vi "Error Interpreter.vi"(0 "request packet":string, 1 "response packet":string, 2 "packet type":T1(ring), 3 "error in (no error)":errorcluster) -> (10 "error out":errorcluster)   [LabVIEW 2024, in "OptoMMP.lvlib"]
doc: "Takes an OptoMMP hexadecimal string formatted response packet of any type, locates the rcode, and outputs a corresponding error code and message. If there is a TCP read error, an Opto error will not be returned.\n\nLast updated: 7/17/2025"
uses:
  <instrlib>/OptoMMP/OptoMMP.lvlib
panel:
  # "Copyright (c) 2025 California Institute of Technology (Caltech).\nU.S. Government sponsorship acknowledged.\n\nLicensed under the Apache License, Version 2.0 (the \"License\");\nyou may not use this file except in compliance with the License.\nYou may obtain a copy of the License at\n\n    http://www.apache.org/licenses/LICENSE-2.0\n\nUnless required by applicable law or agreed to in writing, software\ndistributed under the License is distributed on an \"AS IS\" BASIS,\nWITHOUT WARRANTIES OR CONDITIONS OF ANY KIND, either express or implied.\nSee the License for the specific language governing permissions and\nlimitations under the License."
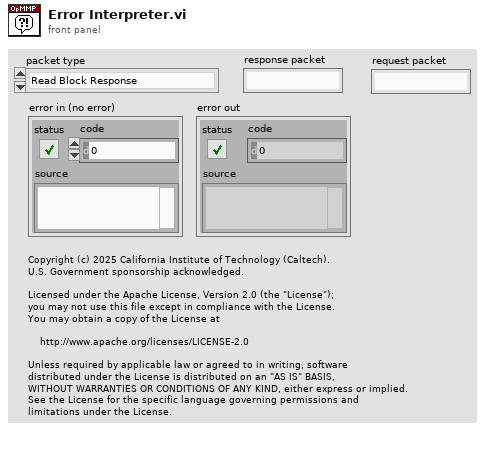
[diagram p1: front panel]
types:
  T1 = enum16{"Read Block Response", "Write Quadlet or Block Response", "Read Quadlet Response"}
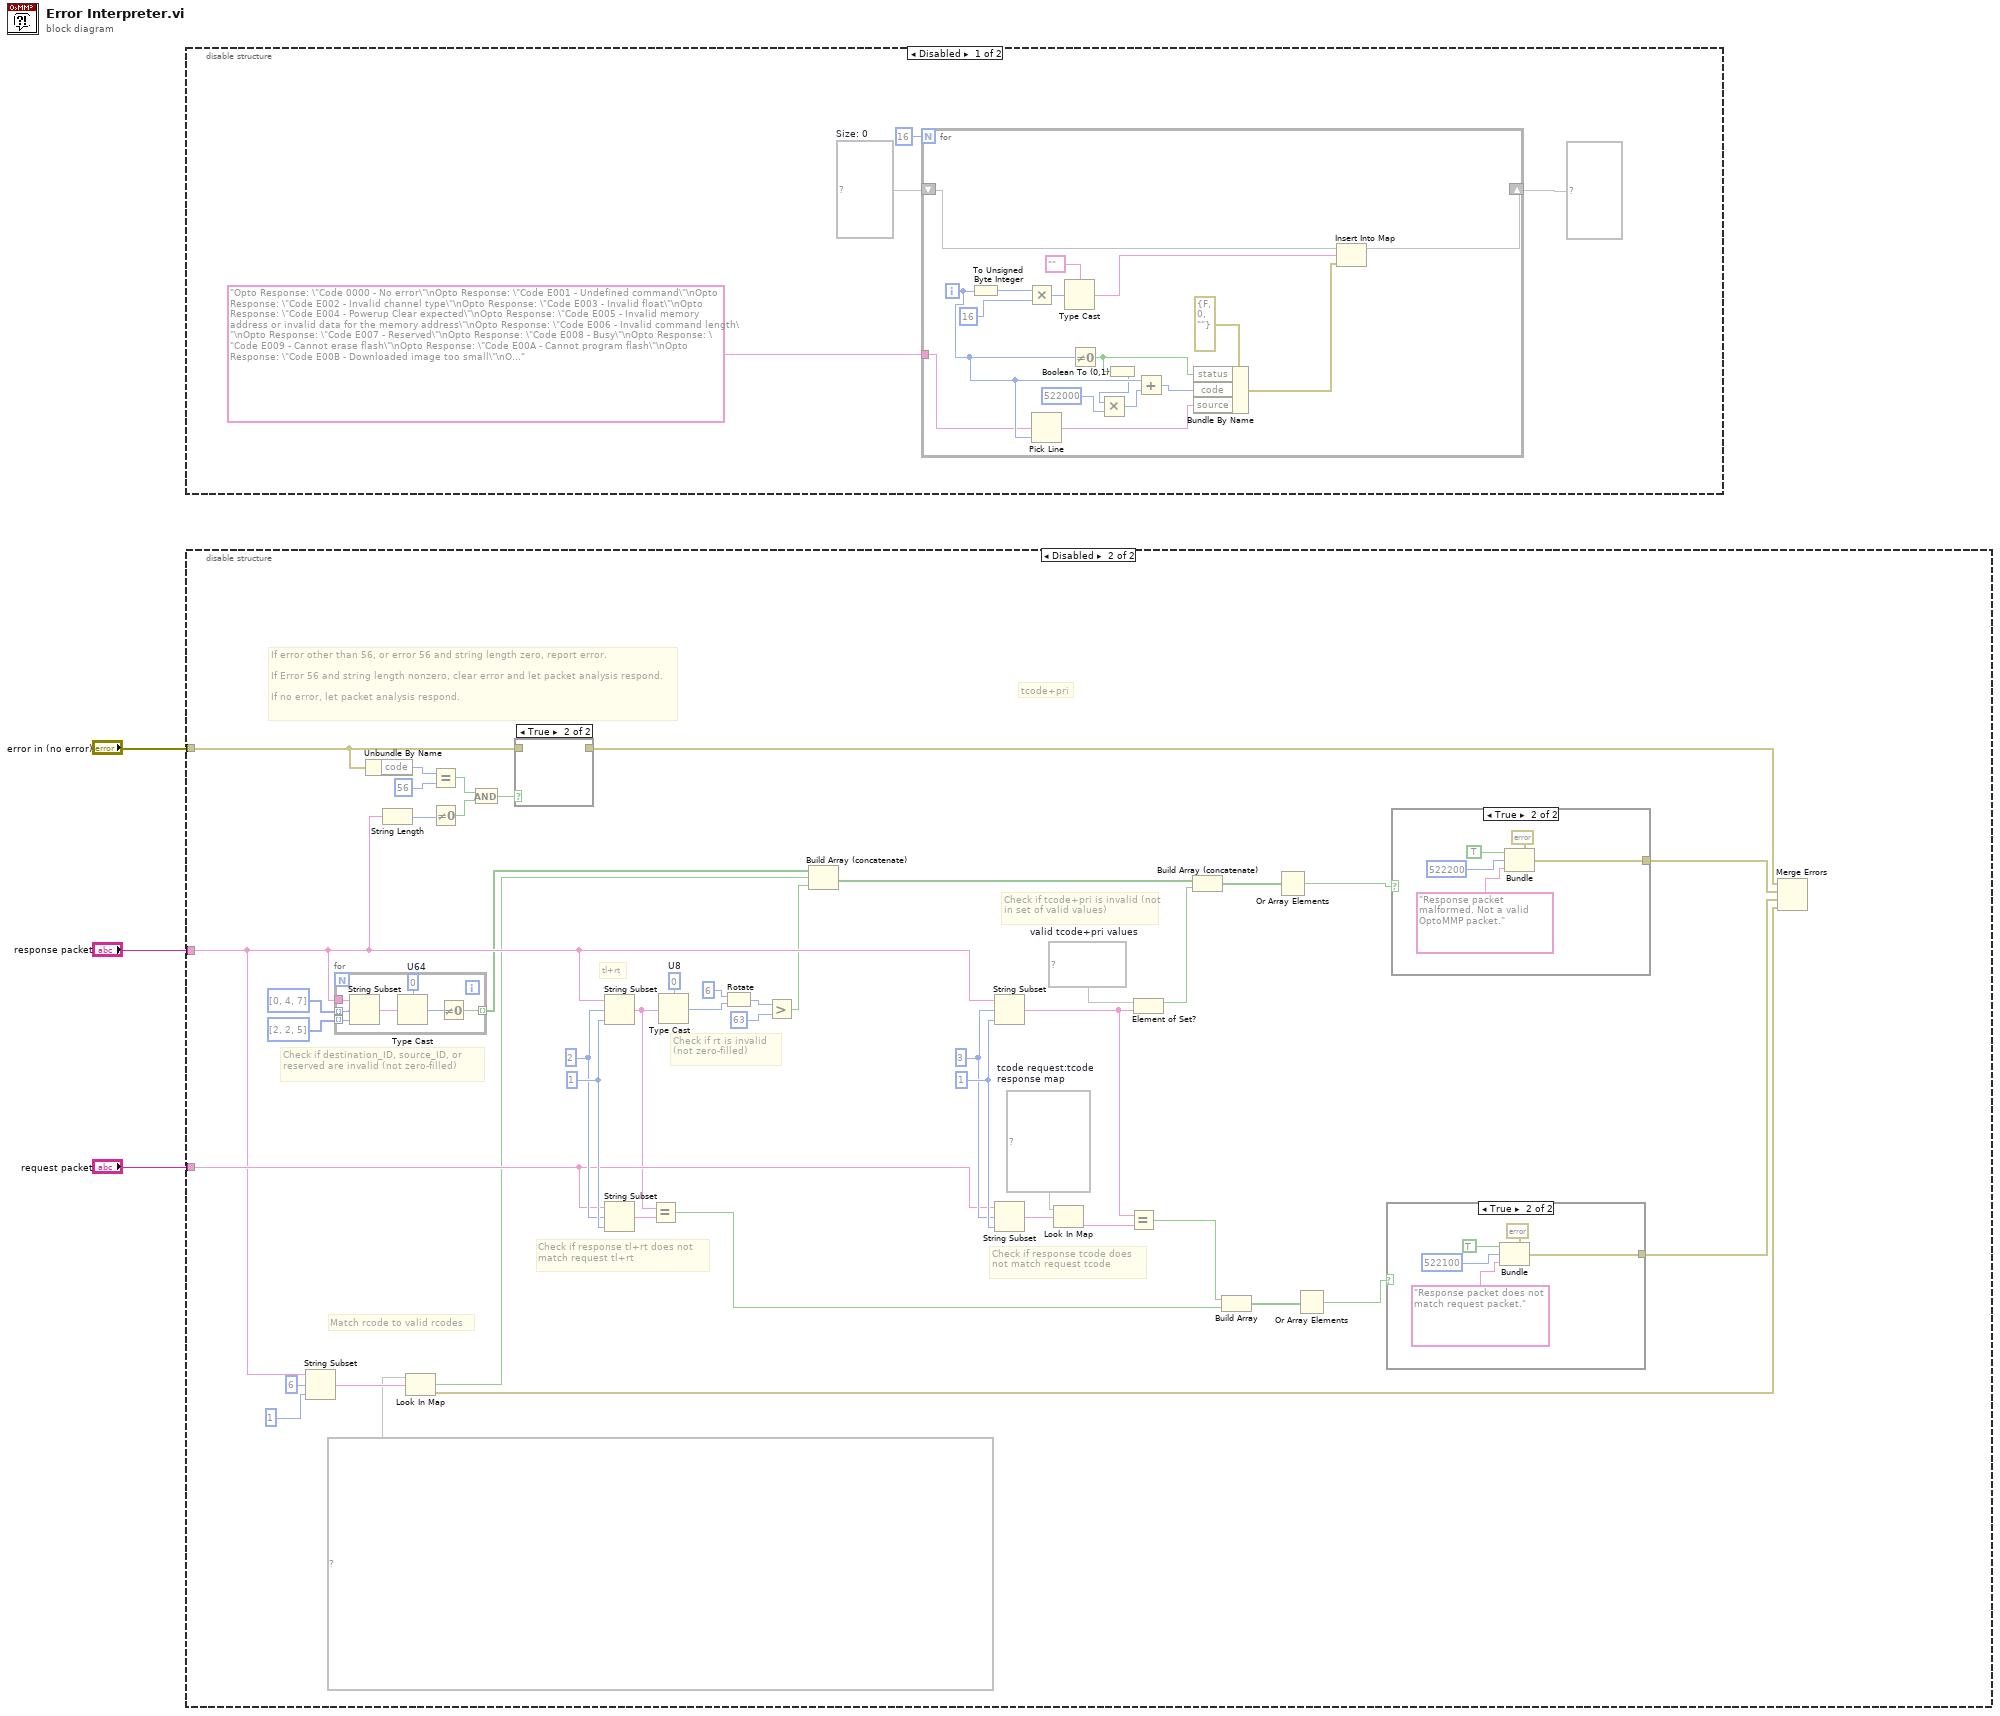
[diagram p0: block diagram]
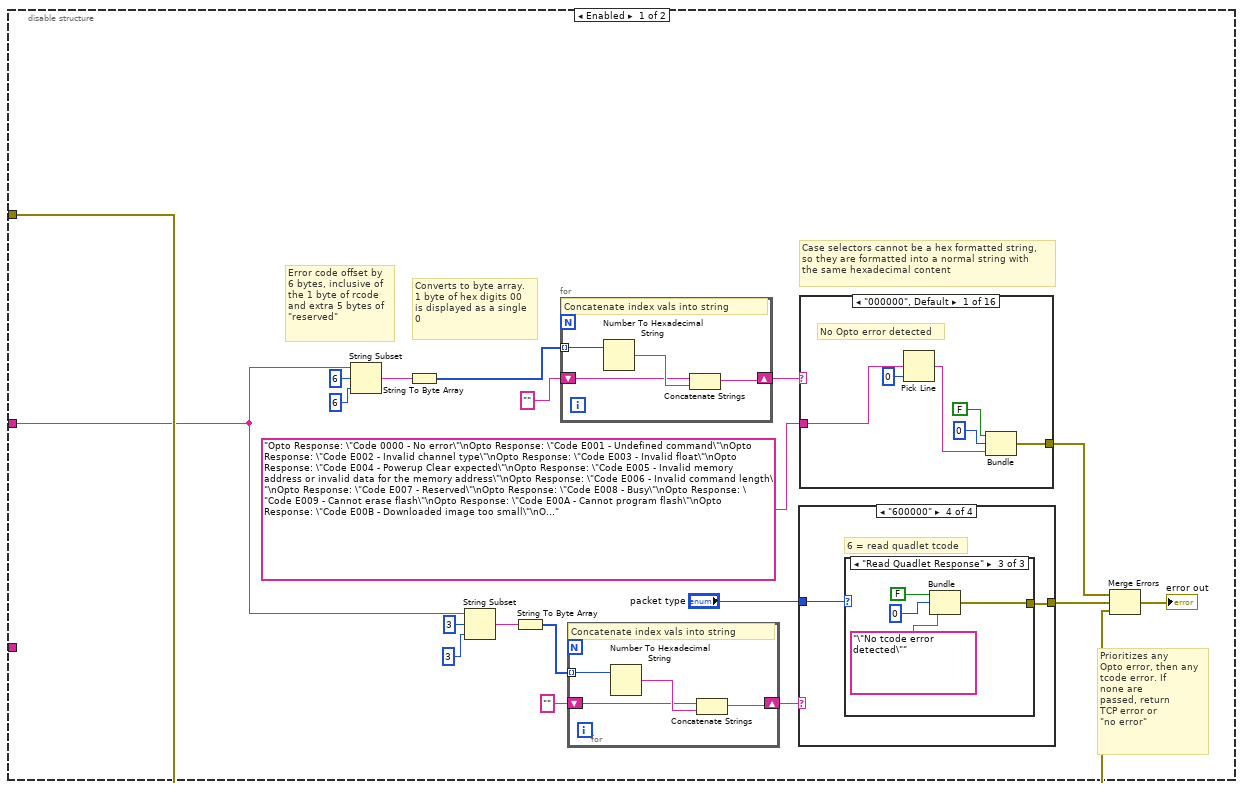
[diagram p3: hidden frame]
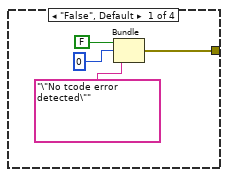
[diagram p4: hidden frame]
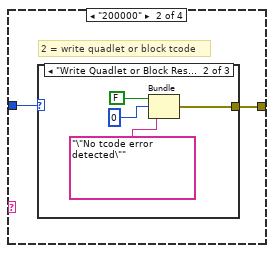
[diagram p5: hidden frame]
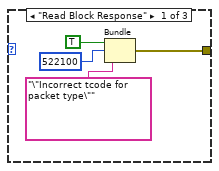
[diagram p6: hidden frame]
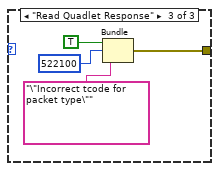
[diagram p7: hidden frame]
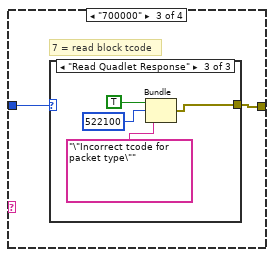
[diagram p8: hidden frame]
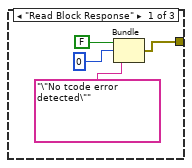
[diagram p9: hidden frame]
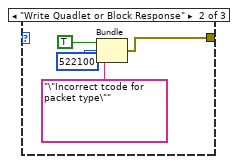
[diagram p10: hidden frame]
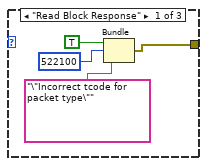
[diagram p11: hidden frame]
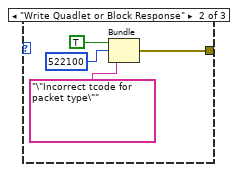
[diagram p12: hidden frame]
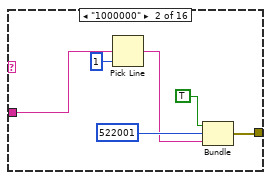
[diagram p13: hidden frame]
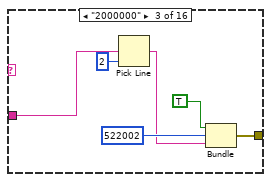
[diagram p14: hidden frame]
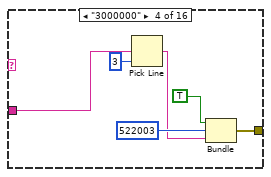
[diagram p15: hidden frame]
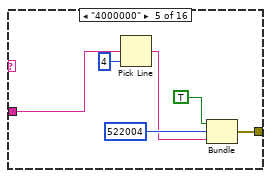
[diagram p16: hidden frame]
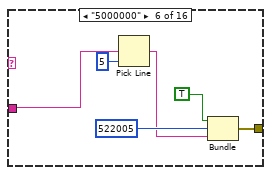
[diagram p17: hidden frame]
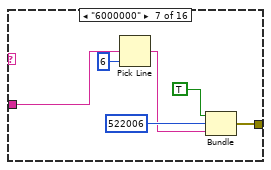
[diagram p18: hidden frame]
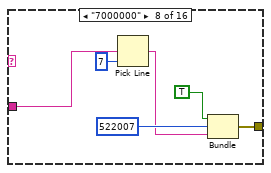
[diagram p19: hidden frame]
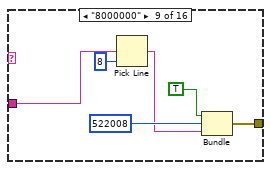
[diagram p20: hidden frame]
diagram:
  n1 = disable-structure shown="Disabled" {
    frame Disabled {
      w4 = map{string, errorcluster} {}  # Size: 0
      n2 = for {
        N: 16 -> [_]
        tunnel: "Opto Response: \"Code 0000 - No error\"\nOpto Response: \"Code E001 - Undefined command\"\nOpto Response: \"Code E002 - Invalid channel type\"\nOpto Response: \"Code E003 - Invalid float\"\nOpto Response: \"Code E004 - Powerup Clear expected\"\nOpto Response: \"Code E005 - Invalid memory address or invalid data for the memory address\"\nOpto Response: \"Code E006 - Invalid command length\"\nOpto Response: \"Code E007 - Reserved\"\nOpto Response: \"Code E008 - Busy\"\nOpto Response: \"Code E009 - Cannot erase flash\"\nOpto Response: \"Code E00A - Cannot program flash\"\nOpto Response: \"Code E00B - Downloaded image too small\"\nOpto Response: \"Code E00C - Image CRC mismatch\"\nOpto Response: \"Code E00D - Image length mismatch\"\nOpto Response: \"Code E00E - Feature is not yet implemented\"\nOpto Response: \"Code E00F - Communications watchdog timeout\"" -> [w14]
        shift-right: [w24] -> w5
        shift-left: w4 -> [w23]
        i -> [w15]
        n3 = To Unsigned Byte Integer(number=w15) -> (unsigned 8bit integer=w21:u8)
        n4 = Multiply(x=w21, y=u8 16) -> (x*y=w20:u8)
        n5 = Pick Line(multi-line string=w14, line index=w15) -> (output string=w13:string)  [unwired: 1 in]
        n6 = Type Cast(type="", x=w20) -> (*(type *) &x=w18:string)
        n7 = Not Equal To 0?(x=w15) -> (x != 0?=w10:bool)
        n8 = Boolean To (0,1)(Boolean=w10) -> (0, 1=w9:i16)
        n9 = Multiply(x=w9, y=522000) -> (x*y=w8:i32)
        n10 = Add(x=w15, y=w8) -> (x+y=w16:i32)
        n11 = Bundle By Name(cluster=errorcluster {"status"=FALSE, "code"=0, "source"=""} ("error constant"), "status"=w10, "code"=w16, "source"=w13) -> (w12:errorcluster)
        n12 = Insert Into Map(map in=w23, key=w18, value=w12) -> (map out=w24:map{string, errorcluster})  [unwired: 2 out]
      }
    }
    frame Enabled {
    }
  }
  n13 = disable-structure shown="Disabled" {
    disable-tunnel: "error in (no error)" -> [w34 w229]
    disable-tunnel: "response packet" -> [w27 w213]
    disable-tunnel: "request packet" -> [_ w221]
    frame Enabled {
      # "Case selectors cannot be a hex formatted string,\nso they are formatted into a normal string with\nthe same hexadecimal content"
      # "Prioritizes any\nOpto error, then any\ntcode error. If\nnone are\npassed, return\nTCP error or\n\"no error\""
      # "Error code offset by\n6 bytes, inclusive of\nthe 1 byte of rcode \nand extra 5 bytes of \n\"reserved\""
      # "Converts to byte array.\n1 byte of hex digits 00\nis displayed as a single\n0"
      n14 = String Subset(string=w27, offset (0)=6, length (rest)=6 ("length (rest)")) -> (substring=w42:string)
      n15 = String To Byte Array(string=w42) -> (unsigned byte array=w40:u8[])
      n16 = String Subset(string=w27, offset (0)=3, length (rest)=3 ("length (rest)")) -> (substring=w30:string)
      n17 = String To Byte Array(string=w30) -> (unsigned byte array=w28:u8[])
      n18 = for {
        tunnel: w40 -> [w97] mode=indexing
        shift-right: [w95] -> w35
        shift-left: "" -> [w94]
        # "Concatenate index vals into string"
        n19 = Number To Hexadecimal String(2:w97) -> (0:w96:string)  [unwired: 1 in]
        n20 = Concatenate Strings(w94, w96) -> (w95:string)
      }
      n21 = for {
        tunnel: w28 -> [w47] mode=indexing
        shift-right: [w45] -> w29
        shift-left: "" -> [w44]
        # "Concatenate index vals into string"
        n22 = Number To Hexadecimal String(2:w47) -> (0:w46:string)  [unwired: 1 in]
        n23 = Concatenate Strings(w44, w46) -> (w45:string)
      }
      n24 = case shown="\"600000\"" w29 {
        tunnel: "packet type" -> [_ w52 w67 w81]
        tunnel: [w48 w53 w66 w80] -> w25
        frame "False", Default {
          n25 = Bundle(FALSE, 0, "\"No tcode error detected\"") -> (w48:errorcluster)  [unwired: 1 in]
        }
        frame "200000" {
          # "2 = write quadlet or block tcode"
          n26 = case shown="\"Write Quadlet or Block Response\"" w52 {
            tunnel: [w54 w58 w62] -> w53
            frame "Read Block Response" {
              n27 = Bundle(TRUE, 522100, "\"Incorrect tcode for packet type\"") -> (w54:errorcluster)  [unwired: 1 in]
            }
            frame "Write Quadlet or Block Response" {
              n28 = Bundle(FALSE, 0, "\"No tcode error detected\"") -> (w58:errorcluster)  [unwired: 1 in]
            }
            frame "Read Quadlet Response" {
              n29 = Bundle(TRUE, 522100, "\"Incorrect tcode for packet type\"") -> (w62:errorcluster)  [unwired: 1 in]
            }
          }
        }
        frame "700000" {
          # "7 = read block tcode"
          n30 = case shown="\"Read Quadlet Response\"" w67 {
            tunnel: [w68 w72 w76] -> w66
            frame "Read Block Response" {
              n31 = Bundle(FALSE, 0, "\"No tcode error detected\"") -> (w68:errorcluster)  [unwired: 1 in]
            }
            frame "Write Quadlet or Block Response" {
              n32 = Bundle(TRUE, 522100, "\"Incorrect tcode for packet type\"") -> (w72:errorcluster)  [unwired: 1 in]
            }
            frame "Read Quadlet Response" {
              n33 = Bundle(TRUE, 522100, "\"Incorrect tcode for packet type\"") -> (w76:errorcluster)  [unwired: 1 in]
            }
          }
        }
        frame "600000" {
          # "6 = read quadlet tcode"
          n34 = case shown="\"Read Quadlet Response\"" w81 {
            tunnel: [w82 w86 w90] -> w80
            frame "Read Block Response" {
              n35 = Bundle(TRUE, 522100, "\"Incorrect tcode for packet type\"") -> (w82:errorcluster)  [unwired: 1 in]
            }
            frame "Write Quadlet or Block Response" {
              n36 = Bundle(TRUE, 522100, "\"Incorrect tcode for packet type\"") -> (w86:errorcluster)  [unwired: 1 in]
            }
            frame "Read Quadlet Response" {
              n37 = Bundle(FALSE, 0, "\"No tcode error detected\"") -> (w90:errorcluster)  [unwired: 1 in]
            }
          }
        }
      }
      n38 = case shown="\"000000\", Default" w35 {
        tunnel: "Opto Response: \"Code 0000 - No error\"\nOpto Response: \"Code E001 - Undefined command\"\nOpto Response: \"Code E002 - Invalid channel type\"\nOpto Response: \"Code E003 - Invalid float\"\nOpto Response: \"Code E004 - Powerup Clear expected\"\nOpto Response: \"Code E005 - Invalid memory address or invalid data for the memory address\"\nOpto Response: \"Code E006 - Invalid command length\"\nOpto Response: \"Code E007 - Reserved\"\nOpto Response: \"Code E008 - Busy\"\nOpto Response: \"Code E009 - Cannot erase flash\"\nOpto Response: \"Code E00A - Cannot program flash\"\nOpto Response: \"Code E00B - Downloaded image too small\"\nOpto Response: \"Code E00C - Image CRC mismatch\"\nOpto Response: \"Code E00D - Image length mismatch\"\nOpto Response: \"Code E00E - Feature is not yet implemented\"\nOpto Response: \"Code E00F - Communications watchdog timeout\"" -> [w98 w108 w114 w120 w126 w132 w138 w144 w150 w156 w162 w168 w174 w180 w186 w192]
        tunnel: [w99 w104 w110 w116 w122 w129 w134 w140 w146 w153 w158 w164 w170 w176 w183 w188] -> w38
        frame "000000", Default {
          # "No Opto error detected"
          n39 = Pick Line(multi-line string=w98, line index=0) -> (output string=w100:string)  [unwired: 1 in]
          n40 = Bundle(FALSE, 0, "output string"=w100) -> (w99:cluster{bool, i32, "output string":string})  [unwired: 1 in]
        }
        frame "1000000" {
          n41 = Pick Line(multi-line string=w108, line index=1) -> (output string=w105:string)  [unwired: 1 in]
          n42 = Bundle(TRUE, 522001, "output string"=w105) -> (w104:cluster{bool, i32, "output string":string})  [unwired: 1 in]
        }
        frame "2000000" {
          n43 = Pick Line(multi-line string=w114, line index=2) -> (output string=w111:string)  [unwired: 1 in]
          n44 = Bundle(TRUE, 522002, "output string"=w111) -> (w110:cluster{bool, i32, "output string":string})  [unwired: 1 in]
        }
        frame "3000000" {
          n45 = Pick Line(multi-line string=w120, line index=3) -> (output string=w117:string)  [unwired: 1 in]
          n46 = Bundle(TRUE, 522003, "output string"=w117) -> (w116:cluster{bool, i32, "output string":string})  [unwired: 1 in]
        }
        frame "4000000" {
          n47 = Pick Line(multi-line string=w126, line index=4) -> (output string=w123:string)  [unwired: 1 in]
          n48 = Bundle(TRUE, 522004, "output string"=w123) -> (w122:cluster{bool, i32, "output string":string})  [unwired: 1 in]
        }
        frame "5000000" {
          n49 = Pick Line(multi-line string=w132, line index=5) -> (output string=w128:string)  [unwired: 1 in]
          n50 = Bundle(TRUE, 522005, "output string"=w128) -> (w129:cluster{bool, i32, "output string":string})  [unwired: 1 in]
        }
        frame "6000000" {
          n51 = Pick Line(multi-line string=w138, line index=6) -> (output string=w135:string)  [unwired: 1 in]
          n52 = Bundle(TRUE, 522006, "output string"=w135) -> (w134:cluster{bool, i32, "output string":string})  [unwired: 1 in]
        }
        frame "7000000" {
          n53 = Pick Line(multi-line string=w144, line index=7) -> (output string=w141:string)  [unwired: 1 in]
          n54 = Bundle(TRUE, 522007, "output string"=w141) -> (w140:cluster{bool, i32, "output string":string})  [unwired: 1 in]
        }
        frame "8000000" {
          n55 = Pick Line(multi-line string=w150, line index=8) -> (output string=w147:string)  [unwired: 1 in]
          n56 = Bundle(TRUE, 522008, "output string"=w147) -> (w146:cluster{bool, i32, "output string":string})  [unwired: 1 in]
        }
        frame "9000000" {
          n57 = Pick Line(multi-line string=w156, line index=9) -> (output string=w152:string)  [unwired: 1 in]
          n58 = Bundle(TRUE, 522009, "output string"=w152) -> (w153:cluster{bool, i32, "output string":string})  [unwired: 1 in]
        }
        frame "A000000" {
          n59 = Pick Line(multi-line string=w162, line index=10) -> (output string=w159:string)  [unwired: 1 in]
          n60 = Bundle(TRUE, 522010, "output string"=w159) -> (w158:cluster{bool, i32, "output string":string})  [unwired: 1 in]
        }
        frame "B000000" {
          n61 = Pick Line(multi-line string=w168, line index=11) -> (output string=w165:string)  [unwired: 1 in]
          n62 = Bundle(TRUE, 522011, "output string"=w165) -> (w164:cluster{bool, i32, "output string":string})  [unwired: 1 in]
        }
        frame "C000000" {
          n63 = Pick Line(multi-line string=w174, line index=12) -> (output string=w171:string)  [unwired: 1 in]
          n64 = Bundle(TRUE, 522012, "output string"=w171) -> (w170:cluster{bool, i32, "output string":string})  [unwired: 1 in]
        }
        frame "D000000" {
          n65 = Pick Line(multi-line string=w180, line index=13) -> (output string=w177:string)  [unwired: 1 in]
          n66 = Bundle(TRUE, 522013, "output string"=w177) -> (w176:cluster{bool, i32, "output string":string})  [unwired: 1 in]
        }
        frame "E000000" {
          n67 = Pick Line(multi-line string=w186, line index=14) -> (output string=w182:string)  [unwired: 1 in]
          n68 = Bundle(TRUE, -522014, "output string"=w182) -> (w183:cluster{bool, i32, "output string":string})  [unwired: 1 in]
        }
        frame "F000000" {
          n69 = Pick Line(multi-line string=w192, line index=15) -> (output string=w189:string)  [unwired: 1 in]
          n70 = Bundle(TRUE, 522015, "output string"=w189) -> (w188:cluster{bool, i32, "output string":string})  [unwired: 1 in]
        }
      }
      n71 = Merge Errors(w38, w25, w34) -> (→"error out":errorcluster)
    }
    frame Disabled {
      w217 = map{string, string} {"\u0000"=" ", "\u0010"=" ", "@"="`", "P"="p"}  # tcode request:tcode response map
      w220 = set{string} {" ", "`", "p"}  # valid tcode+pri values
      w223 = 1 ("length (rest)")
      w222 = 3 ("offset (0)")
      w228 = u8 0  # U8
      w237 = 1 ("length (rest)")
      w236 = 2 ("offset (0)")
      # "Match rcode to valid rcodes"
      # "Check if response tcode does not match request tcode"
      # "Check if response tl+rt does not match request tl+rt"
      # "Check if tcode+pri is invalid (not in set of valid values)"
      # "Check if rt is invalid (not zero-filled)"
      # "Check if destination_ID, source_ID, or reserved are invalid (not zero-filled)"
      # "tcode+pri"
      # "tl+rt"
      # "If error other than 56, or error 56 and string length zero, report error.\n\nIf Error 56 and string length nonzero, clear error and let packet analysis respond.\n\nIf no error, let packet analysis respond."
      n72 = String Subset(string=w213, offset (0)=6, length (rest)=1 ("length (rest)")) -> (substring=w210:string)
      n73 = for {
        tunnel: w213 -> [w257]
        tunnel: i32[] [0, 4, 7] -> [w256] mode=indexing
        tunnel: i32[] [2, 2, 5] -> [w255] mode=indexing
        tunnel: [w251] -> w207 mode=indexing
        w254 = u64 0  # U64
        n74 = String Subset(string=w257, offset (0)=w256, length (rest)=w255) -> (substring=w253:string)
        n75 = Type Cast(type=w254, x=w253) -> (*(type *) &x=w252:u64)
        n76 = Not Equal To 0?(x=w252) -> (x != 0?=w251:bool)
      }
      n77 = Unbundle By Name(w229) -> ("code"=w235:i32)
      n78 = String Length(string=w213) -> (length=w233:i32)
      n79 = Look In Map(map=map{string, errorcluster} {"\u0000"={"status"=FALSE, "code"=0, "source"="Opto Response: \"Code 0000 - No error\""}, "\u0010"={"status"=TRUE, "code"=522001, "source"="Opto Response: \"Code E001 - Undefined command\""}, " "={"status"=TRUE, "code"=522002, "source"="Opto Response: \"Code E002 - Invalid channel type\""}, "0"={"status"=TRUE, "code"=522003, "source"="Opto Response: \"Code E003 - Invalid float\""}, "@"={"status"=TRUE, "code"=522004, "source"="Opto Response: \"Code E004 - Powerup Clear expected\""}, "P"={"status"=TRUE, "code"=522005, "source"="Opto Response: \"Code E005 - Invalid memory address or invalid data for the memory address\""}, "`"={"status"=TRUE, "code"=522006, "source"="Opto Response: \"Code E006 - Invalid command length\""}, "p"={"status"=TRUE, "code"=522007, "source"="Opto Response: \"Code E007 - Reserved\""}, "€"={"status"=TRUE, "code"=522008, "source"="Opto Response: \"Code E008 - Busy\""}, ""={"status"=TRUE, "code"=522009, "source"="Opto Response: \"Code E009 - Cannot erase flash\""}, " "={"status"=TRUE, "code"=522010, "source"="Opto Response: \"Code E00A - Cannot program flash\""}, "°"={"status"=TRUE, "code"=522011, "source"="Opto Response: \"Code E00B - Downloaded image too small\""}, "À"={"status"=TRUE, "code"=522012, "source"="Opto Response: \"Code E00C - Image CRC mismatch\""}, "Ð"={"status"=TRUE, "code"=522013, "source"="Opto Response: \"Code E00D - Image length mismatch\""}, "à"={"status"=TRUE, "code"=522014, "source"="Opto Response: \"Code E00E - Feature is not yet implemented\""}, "ð"={"status"=TRUE, "code"=522015, "source"="Opto Response: \"Code E00F - Communications watchdog timeout\""}} ("Map"), key=w210) -> (key not found?=w205:bool, value=w194:errorcluster)  [unwired: 1 in]
      n80 = Equal?(x=w235, y=56) -> (x = y?=w232:bool)
      n81 = Not Equal To 0?(x=w233) -> (x != 0?=w231:bool)
      n82 = And(x=w232, y=w231) -> (x .and. y?=w230:bool)
      n83 = case shown="True" w230 {
        tunnel: w229 -> [w250 _]
        tunnel: [w250 _] -> w199
        frame False {
        }
        frame True {
        }
      }
      n84 = String Subset(string=w213, offset (0)=w236, length (rest)=w237) -> (substring=w218:string)
      n85 = String Subset(string=w221, offset (0)=w236, length (rest)=w237) -> (substring=w219:string)
      n86 = Equal?(x=w218, y=w219) -> (x = y?=w208:bool)
      n87 = Type Cast(type=w228, x=w218) -> (*(type *) &x=w227:u8)
      n88 = Rotate(1:w227, 2:i16 6 ("y")) -> (0:w225:u8)
      n89 = Greater?(x=w225, y=u8 63) -> (0:w206:bool)
      n90 = Build Array (concatenate)(w207, w205, w206) -> (w204:bool[])
      n91 = String Subset(string=w213, offset (0)=w222, length (rest)=w223) -> (substring=w215:string)
      n92 = String Subset(string=w221, offset (0)=w222, length (rest)=w223) -> (substring=w216:string)
      n93 = Look In Map(map=w217, key=w216) -> (value=w214:string)  [unwired: 1 in, 1 out]
      n94 = Equal?(x=w215, y=w214) -> (x = y?=w198:bool)
      n95 = Element of Set?(10:w215, 11:w220) -> (3:w203:bool)
      n96 = Build Array (concatenate)(w204, w203) -> (w202:bool[])
      n97 = Build Array(w198, w208) -> (w197:bool[])
      n98 = Or Array Elements(Boolean array=w202) -> (logical OR=w201:bool)
      n99 = Or Array Elements(Boolean array=w197) -> (logical OR=w196:bool)
      n100 = case shown="True" w196 {
        tunnel: [_ w240] -> w195
        frame False {
        }
        frame True {
          n101 = Bundle(cluster=errorcluster {FALSE, 0, ""}, TRUE, 522100, "Response packet does not match request packet.") -> (w240:errorcluster)
        }
      }
      n102 = case shown="True" w201 {
        tunnel: [_ w245] -> w200
        frame False {
        }
        frame True {
          n103 = Bundle(cluster=errorcluster {FALSE, 0, ""}, TRUE, 522200, "Response packet malformed. Not a valid OptoMMP packet.") -> (w245:errorcluster)
        }
      }
      n104 = Merge Errors(w199, w200, w195, w194) -> ()  [unwired: 1 out]
    }
  }
